vi "DetectorReadData-1D.vi"(0 "Microscope in":refnum<class "Microscope.lvclass">, 1 "Detector Type":T1, 3 "Actual Samples Per Line":i32, 4 "Computed Parameter.Samples to Average":i32, 5 "Computed Parameter.Trash Samples":i32, 7 "Hardware Settings.Digital Image Multiplier":dbl=100.0, 9 "error in (no error)":errorcluster, 11 "show flyback data":bool, 13 "disable averaging":bool) -> (14 "Microscope out":refnum<class "Microscope.lvclass">, 15 "Data":dbl[][](array[numeric]), 19 "error out":errorcluster)   [LabVIEW 2012, in "Microscope.lvclass"]
uses:
  classes/Microscope.lvclass
  typedefs/DetectorType.ctl
  classes/Microscope.lvclass/Microscope.ctl
  <vilib>/DAQmx/read.llb/DAQmx Read (Analog 2D DBL NChan NSamp).vi
  <vilib>/DAQmx/miscellaneous.llb/DAQmx Fill In Error Info.vi
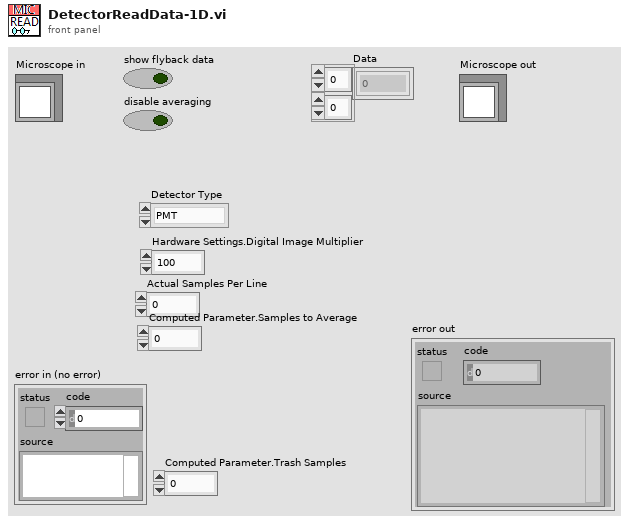
[diagram p1: front panel]
types:
  T1 = typedef "DetectorType.ctl" = enum16{"PMT", "SpectraWiz"}
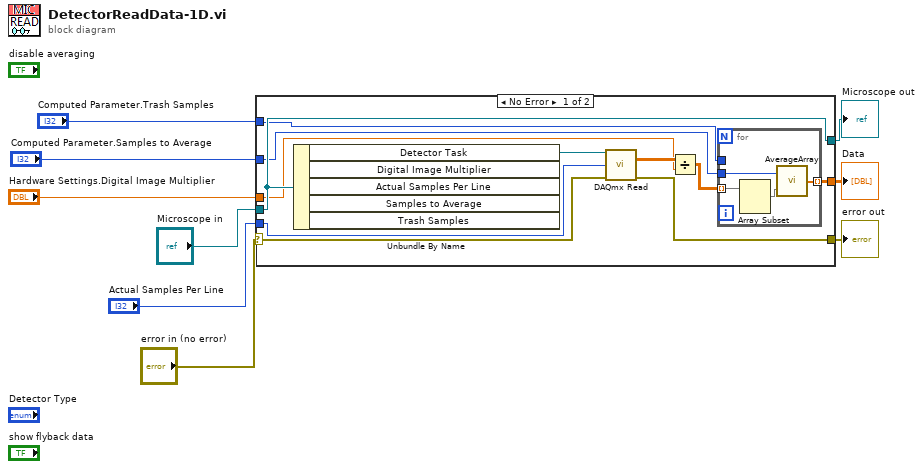
[diagram p0: block diagram]
diagram:
  n1 = case shown="No Error" "error in (no error)" {
    selector: "error in (no error)" -> [w14 w26]
    tunnel: [w16 w26] -> w8
    tunnel: [w15 w25] -> w6
    tunnel: "Microscope in" -> [w15 w25]
    tunnel: [w19 _] -> w5
    tunnel: "Hardware Settings.Digital Image Multiplier" -> [w13 _]
    tunnel: "Computed Parameter.Samples to Average" -> [w12 _]
    tunnel: "Computed Parameter.Trash Samples" -> [w11 _]
    tunnel: "Actual Samples Per Line" -> [w10 _]
    frame No Error {
      n2 = Unbundle By Name(w15) -> ("Detector Task"=w20:refnum<k21>)  [unwired: 4 out]
      n3 = call-poly <vilib>:"DAQmx Read.vi"("task/channels in"=w20, "number of samples per channel"=w10, "error in"=w14) -> ("data"=w18:dbl[][], "error out"=w16:errorcluster)  [unwired: 10 in, 1 out]
      n4 = Divide(x=w18, y=w13) -> (x/y=w17:dbl[][])
      n5 = for {
        tunnel: w17 -> [w23] mode=indexing
        tunnel: w12 -> [w22]
        tunnel: w11 -> [_]
        tunnel: [w21] -> w19 mode=indexing
        n6 = Array Subset(array=w23) -> (w24:dbl[])  [unwired: 2 in]
        n7 = call "AverageArray.vi"("Input Array"=w24, "Samples To Average"=w22) -> ("Averaged Array"=w21:dbl[])
      }
    }
    frame Error {
    }
  }
  "error out" <- w8
  "Microscope out" <- w6
  "Data" <- w5
